vi "AccelerometerTest.vi"() -> ()   [LabVIEW 2016]
uses:
  <vilib>/rvi/interface/nirviOpenFPGA/nirviOpenFPGA.xnode
  <vilib>/rvi/interface/nirviMethod/nirviMethod.xnode
  <vilib>/FPGAPlugInAG/Dynamic/niLvFpga_Abort_Dynamic.vi
  <vilib>/FPGAPlugInAG/Dynamic/niLvFpga_Run_Dynamic.vi
  <vilib>/rvi/interface/nirviCloseFPGA/nirviCloseFPGA.xnode
  <vilib>/FPGAPlugInAG/Dynamic/niLvFpga_Reset_Dynamic.vi
  <vilib>/Platform/TimedLoop/XDataNode/XDataNode.xnode
  <vilib>/Platform/TimedLoop/XDataNode/nitl_modes.ctl
  <vilib>/Platform/TimedLoop/XDataNode/XDNodeRunTimeDep.lvlib
  <vilib>/Platform/TimedLoop/XDataNode/wakeup.ctl
  <vilib>/Platform/TimedLoop/XDataNode/timing_clust.ctl
  Accel1TimestampFIFO/Accel1TimestampFIFO.lvclass
  Scratch/RTMonitorAccelerometer/MonitorAccelerometer/MonitorAccelerometer.lvclass
  Accel1Channel0FIFO/Accel1Channel0FIFO.lvclass
  Accel1Channel1FIFO/Accel1Channel1FIFO.lvclass
  Accel1Channel2FIFO/Accel1Channel2FIFO.lvclass
  AccelCommandFIFO/AccelCommandFIFO.lvclass
  FPGA Bitfiles/modbus1Port.lvbitx
  FPGA/main.vi
  <vilib>/FPGAPlugInAG/cRIO-9038/niLvFpga_Open_cRIO-9038.vi
  <vilib>/rvi/interface/common/dynamic/niFpgaDynamicAddResources.vi
  <vilib>/FPGAPlugInAG/Dynamic/niLvFpga_Close_Dynamic.vi
  D:/Code/Common_RT_FPGA/IReadU64FIFO/IReadU64FIFO.lvclass
  D:/Code/Common_RT_FPGA/IReadSGLFIFO/IReadSGLFIFO.lvclass
  D:/Code/Common_RT_FPGA/IWriteU32FIFO/IWriteU32FIFO.lvclass
panel:
  in  "Boolean":bool
  in  "PeriodInMicroseconds":u32=1000
  out "Accelerometer":cluster{"Timestamp":dbl[], "Channel2":sgl[]}[](graph)
  out "error out":errorcluster
  # "Port 1 = Modbus"
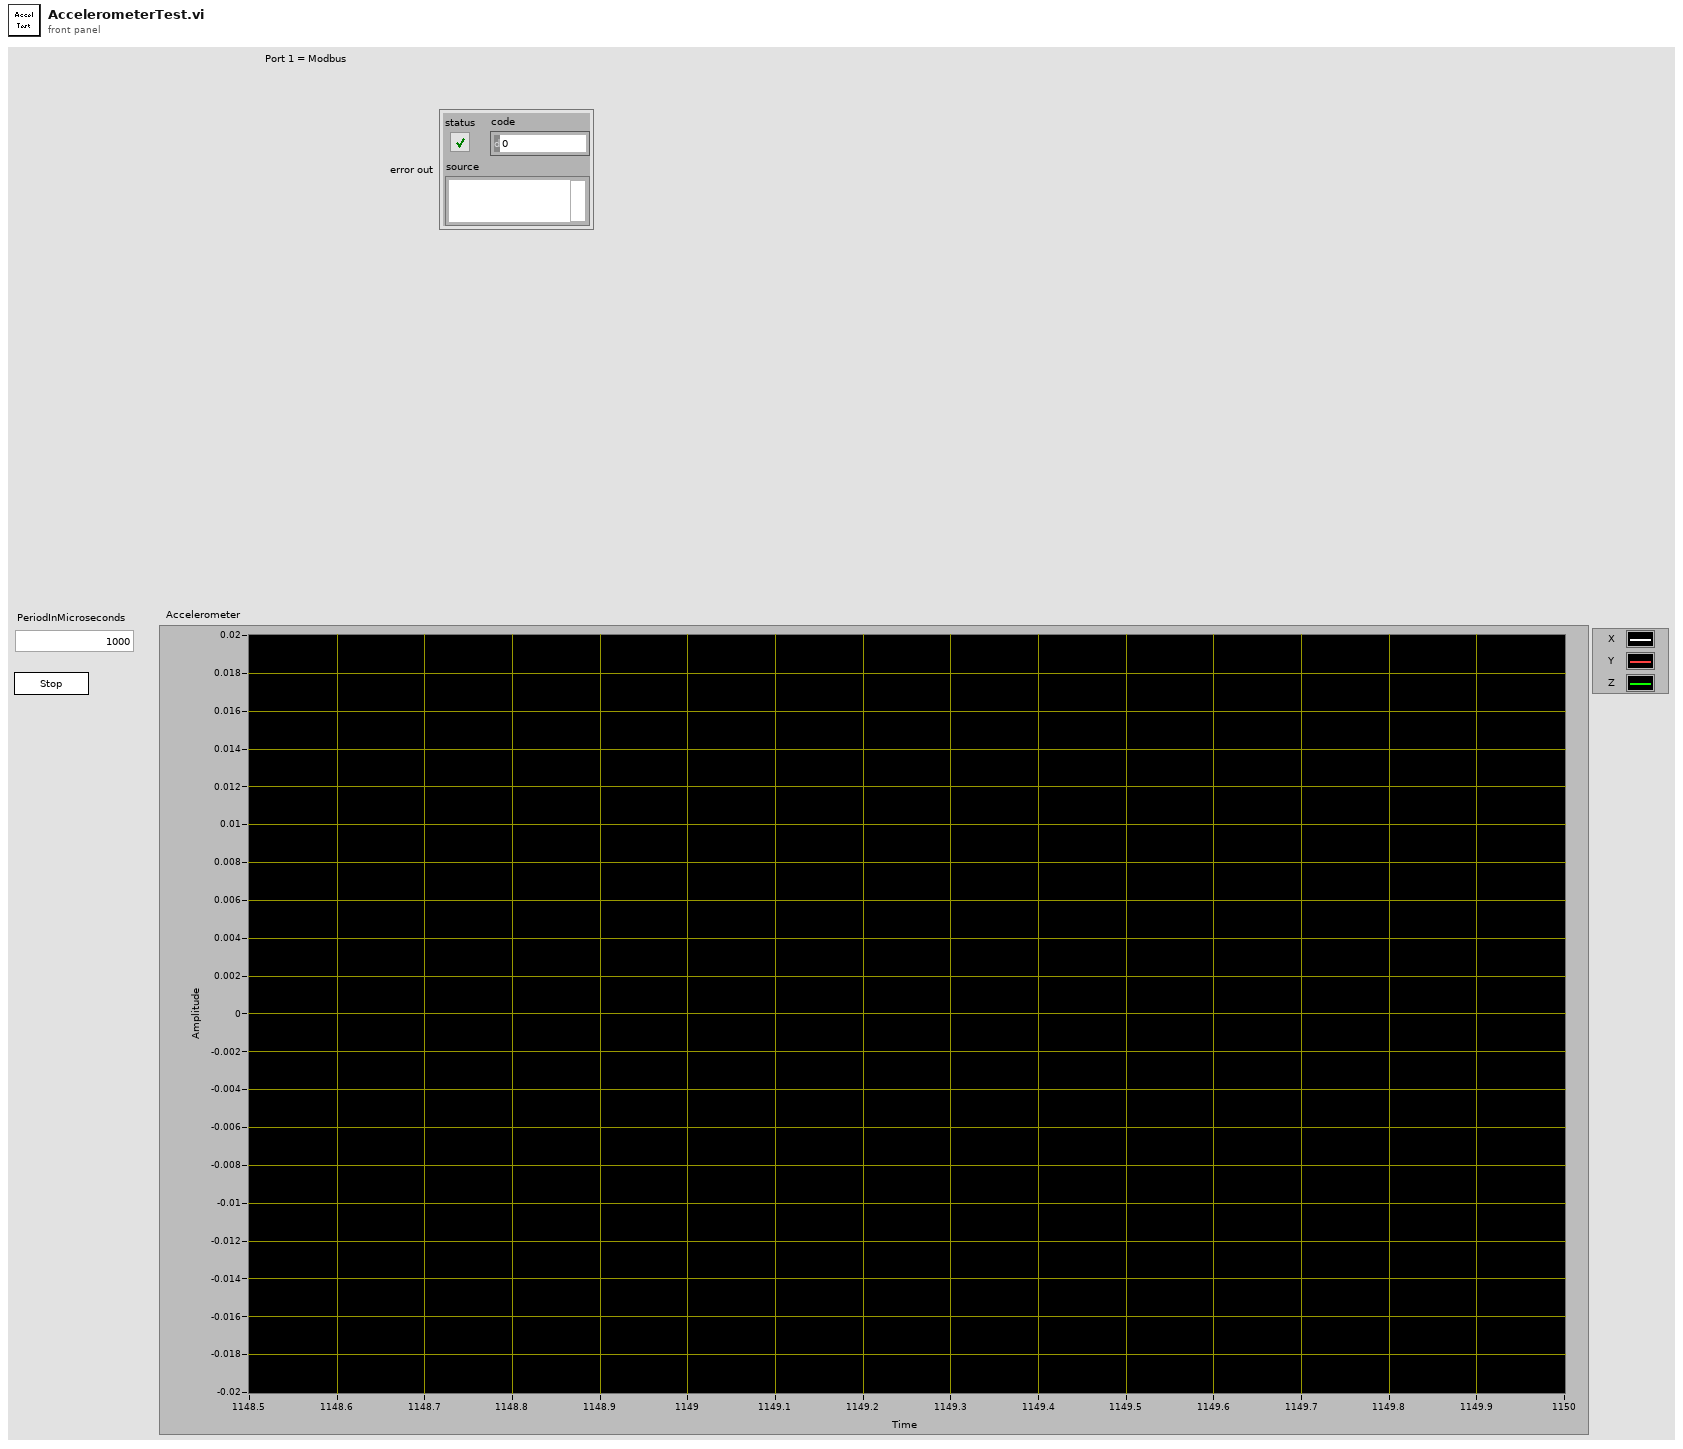
[diagram p1: front panel]
types:
  T1 = typedef "XDNodeRunTimeDep.lvlib/timing_clust.ctl" = cluster{"Expected End [f-1]":u64, "Actual End [f-1]":u64, "Finished Late? [f-1]":bool, "Expected End [i-1]":u64, "Actual End [i-1]":u64, "Finished Late? [i-1]":bool, "Expected Start [i]":u64, "Actual Start [i]":u64, "Expected Start [f]":u64, "Actual Start [f]":u64, "Source Name":string, "Structure Name":string, "Period":i64, "Deadline":i64, "Offset":i64, "Start":i64, "Priority":i32, "Timeout":i32, "Mode":T2, "Wakeup Reason":T3, "Error":errorcluster, "Source Type":string, "Secondary Source Type":string, "Global End Time":u64, "Global Start Time":u64, "Frame Duration":u64, "Iteration Duration":u64, "Assigned CPU":i32, "I/O Scan Engine Mode":u32}
  T2 = typedef "XDNodeRunTimeDep.lvlib/nitl_modes.ctl" = enum32{"No Change", "Process missed periods, maintain original phase", "Discard missed periods, maintain original phase", "Process missed periods, ignore original phase", "Discard missed periods, ignore original phase"}
  T3 = typedef "XDNodeRunTimeDep.lvlib/wakeup.ctl" = enum32{"Normal", "Aborted", "Asynchronous wakeup", "Timing source error", "Timed loop error", "Timeout"}
  T4 = typedef "RTMonitorAccelerometer.lvlib/MonitorAccelerometerData.ctl" = cluster{"Timestamp":dbl[], "Channel0":sgl[], "Channel1":sgl[], "Channel2":sgl[]}
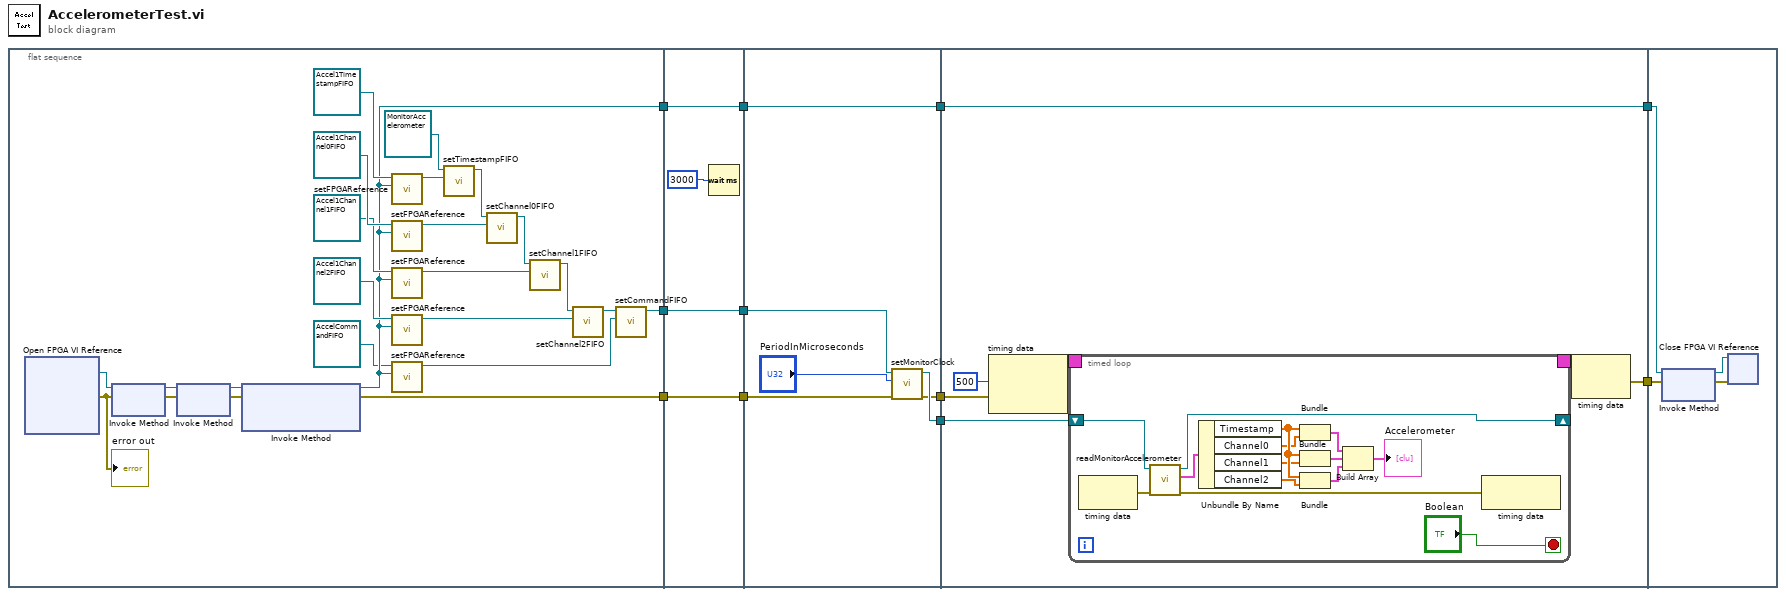
[diagram p0: block diagram]
diagram:
  n1 = flat-sequence {
    tunnel: [w12] -> w6
    tunnel: [w16] -> w4
    tunnel: [w17] -> w2
    tunnel: w6 -> [w39]
    tunnel: [w39] -> w5
    tunnel: w4 -> [w38]
    tunnel: [w38] -> w3
    tunnel: w2 -> [w37]
    tunnel: [w37] -> w1
    tunnel: w5 -> [w44]
    tunnel: [w43] -> w11
    tunnel: [w45] -> w9
    tunnel: w3 -> [w45]
    tunnel: w1 -> [w41]
    tunnel: [w40] -> w8
    tunnel: w11 -> [w49]
    tunnel: [w48] -> w10
    tunnel: w9 -> [w48]
    tunnel: w8 -> [w47]
    tunnel: [w46] -> w7
    tunnel: w10 -> [w80]
    tunnel: w7 -> [w79]
    frame #0 {
      n2 = xnode "Open FPGA VI Reference"() -> ("FPGA VI Reference Out"=w33:refnum<k20>, "error out"=w30:errorcluster)  [unwired: 2 in]
      "error out" <- w30
      n3 = xnode "Invoke Method"("FPGA VI Reference In"=w33, "error in"=w30) -> ("FPGA VI Reference Out"=w35:refnum<k20>, "error out"=w34:errorcluster)
      n4 = xnode "Invoke Method"("FPGA VI Reference In"=w35, "error in"=w34) -> ("FPGA VI Reference Out"=w32:refnum<k20>, "error out"=w31:errorcluster)
      n5 = xnode "Invoke Method"("FPGA VI Reference In"=w32, "error in"=w31) -> ("FPGA VI Reference Out"=w16:refnum<k20>, "error out"=w17:errorcluster)  [unwired: 1 in]
      n6 = call "setFPGAReference.vi"("FPGAReference"=w16, "MyHealthAndStatusReadFIFO in"=refnum<class "Accel1TimestampFIFO.lvclass"> refnum ("Accel1TimestampFIFO.lvclass")) -> ("MyHealthAndStatusReadFIFO out"=w26:refnum<class "Accel1TimestampFIFO.lvclass">)  [unwired: 9 in]
      n7 = call "setFPGAReference.vi"("FPGAReference"=w16, "MyHealthAndStatusReadFIFO in"=refnum<class "Accel1Channel0FIFO.lvclass"> refnum ("Accel1Channel0FIFO.lvclass")) -> ("MyHealthAndStatusReadFIFO out"=w22:refnum<class "Accel1Channel0FIFO.lvclass">)  [unwired: 9 in]
      n8 = call "setFPGAReference.vi"("FPGAReference"=w16, "MyHealthAndStatusReadFIFO in"=refnum<class "Accel1Channel1FIFO.lvclass"> refnum ("Accel1Channel1FIFO.lvclass")) -> ("MyHealthAndStatusReadFIFO out"=w20:refnum<class "Accel1Channel1FIFO.lvclass">)  [unwired: 9 in]
      n9 = call "setFPGAReference.vi"("FPGAReference"=w16, "MyHealthAndStatusReadFIFO in"=refnum<class "Accel1Channel2FIFO.lvclass"> refnum ("Accel1Channel2FIFO.lvclass")) -> ("MyHealthAndStatusReadFIFO out"=w18:refnum<class "Accel1Channel2FIFO.lvclass">)  [unwired: 9 in]
      n10 = call "setFPGAReference.vi"("FPGAReference"=w16, "ModbusPort1WriteFIFO in"=refnum<class "AccelCommandFIFO.lvclass"> refnum ("AccelCommandFIFO.lvclass")) -> ("ModbusPort1WriteFIFO out"=w14:refnum<class "AccelCommandFIFO.lvclass">)  [unwired: 9 in]
      n11 = call "setTimestampFIFO.vi"("TimestampFIFO"=w26, "MonitorAccelerometer in"=refnum<class "MonitorAccelerometer.lvclass"> refnum ("RTMonitorAccelerometer.lvlib:MonitorAccelerometer.lvclass")) -> ("MonitorAccelerometer out"=w27:refnum<class "MonitorAccelerometer.lvclass">)  [unwired: 9 in]
      n12 = call "setChannel0FIFO.vi"("Channel0FIFO"=w22, "MonitorAccelerometer in"=w27) -> ("MonitorAccelerometer out"=w25:refnum<class "MonitorAccelerometer.lvclass">)  [unwired: 9 in]
      n13 = call "setChannel1FIFO.vi"("Channel1FIFO"=w20, "MonitorAccelerometer in"=w25) -> ("MonitorAccelerometer out"=w24:refnum<class "MonitorAccelerometer.lvclass">)  [unwired: 9 in]
      n14 = call "setChannel2FIFO.vi"("Channel2FIFO"=w18, "MonitorAccelerometer in"=w24) -> ("MonitorAccelerometer out"=w13:refnum<class "MonitorAccelerometer.lvclass">)  [unwired: 9 in]
      n15 = call "setCommandFIFO.vi"("CommandFIFO"=w14, "MonitorAccelerometer in"=w13) -> ("MonitorAccelerometer out"=w12:refnum<class "MonitorAccelerometer.lvclass">)  [unwired: 9 in]
    }
    frame #1 {
      n16 = Wait (ms)(milliseconds to wait=u32 3000) -> ()  [unwired: 1 out]
    }
    frame #2 {
      n17 = call "setMonitorClock.vi"("error in (no error)"=w41, "PeriodInMicroseconds"="PeriodInMicroseconds", "MonitorAccelerometer in"=w44) -> ("error out"=w40:errorcluster, "MonitorAccelerometer out"=w43:refnum<class "MonitorAccelerometer.lvclass">)  [unwired: 7 in]
    }
    frame #3 {
      n18 = node-c288(i64 500 ("Period"), w47) -> (w52:T1)
      n19 = timed-loop {
        timing: w52 -> [_]
        timing-out: [_] -> w51
        shift-right: [w65] -> _
        shift-left: w49 -> [w66]
        stop <- "Boolean" stop-if-true
        n20 = node-c288() -> (w54:errorcluster)  [unwired: 1 in]
        n21 = call "readMonitorAccelerometer.vi"("error in (no error)"=w54, "MonitorAccelerometer in"=w66) -> ("error out"=w53:errorcluster, "MonitorAccelerometerData"=w60:T4, "MonitorAccelerometer out"=w65:refnum<class "MonitorAccelerometer.lvclass">)  [unwired: 7 in]
        n22 = Unbundle By Name(w60) -> ("Timestamp"=w64:dbl[], "Channel0"=w63:sgl[], "Channel1"=w62:sgl[], "Channel2"=w61:sgl[])
        n23 = Bundle("Timestamp"=w64, "Channel0"=w63) -> (w59:cluster{"Timestamp":dbl[], "Channel0":sgl[]})  [unwired: 1 in]
        n24 = Bundle("Timestamp"=w64, "Channel1"=w62) -> (w58:cluster{"Timestamp":dbl[], "Channel1":sgl[]})  [unwired: 1 in]
        n25 = Bundle("Timestamp"=w64, "Channel2"=w61) -> (w57:cluster{"Timestamp":dbl[], "Channel2":sgl[]})  [unwired: 1 in]
        n26 = Build Array(w59, w58, w57) -> (→"Accelerometer":cluster{"Timestamp":dbl[], "Channel2":sgl[]}[])
        n27 = node-c288(w53) -> ()  [unwired: 1 out]
      }
      n28 = node-c288(w51) -> (w46:errorcluster)
    }
    frame #4 {
      n29 = xnode "Invoke Method"("FPGA VI Reference In"=w80, "error in"=w79) -> ("FPGA VI Reference Out"=w81:refnum<k20>, "error out"=w78:errorcluster)
      n30 = xnode "Close FPGA VI Reference"("FPGA VI Reference In"=w81, "error in"=w78) -> ()  [unwired: 1 out]
    }
  }
